vi "SecOverlayParams.vi"(4 "Scan Info":T1, 6 "Time between rf pts\nmicros":dbl, 7 "pixels in y":i16, 9 "c m/s":dbl=1500.0, 10 "Array":i32[](array[numeric]), 11 "pixels in x":i16) -> (0 "scales":cluster{"inc x (mm)":dbl, "inc y (mm)":dbl}, 1 "y scaled":dbl[][](array[numeric]), 2 "x scaled":dbl[][](array[numeric]), 3 "Axis scaling Params":T2 {"Y high" format="%.2f"; "Y low" format="%.2f"; "X left" format="%.2f"; "X right" format="%.2f"})   [LabVIEW 2022 SP3]
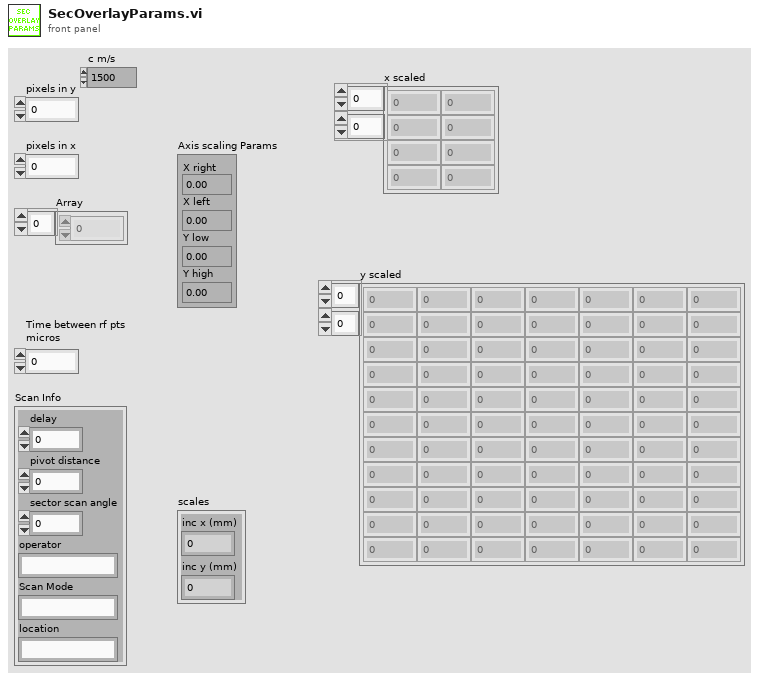
[diagram p1: front panel]
types:
  T1 = cluster{"delay":sgl, "pivot distance":sgl, "sector scan angle":sgl, "operator":string, "Scan Mode":string, "location":string}
  T2 = cluster{"X right":dbl, "X left":dbl, "Y low":dbl, "Y high":dbl}
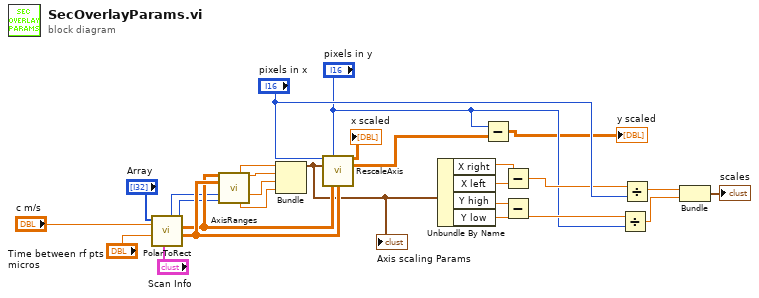
[diagram p0: block diagram]
diagram:
  n1 = call "PolarToRect.vi"("Scan Info"="Scan Info", "Time between pt\nmicros"="Time between rf pts\nmicros", "c m/s"="c m/s", "array dims"="Array") -> ("y"=w9:dbl[][], "x"=w8:dbl[][], "# lines per scan"=w7:u16, "# rf points per line"=w6:u16)  [unwired: 4 out]
  n2 = call "AxisRanges.vi"("x"=w8, "y"=w9, "# rf points per line"=w6, "# lines per scan"=w7) -> ("X right"=w10:dbl, "X left"=w13:dbl, "Y low"=w11:dbl, "Y high"=w12:dbl)  [unwired: 1 in, 7 out]
  n3 = Bundle("X right"=w10, "X left"=w13, "Y low"=w11, "Y high"=w12) -> (w5:T2)  [unwired: 1 out]
  "Axis scaling Params" <- w5
  n4 = call "RescaleAxis.vi"("pixels in x"="pixels in x", "pixels in y"="pixels in y", "Axis scaling Params"=w5, "x"=w8, "y"=w9) -> ("x scaled"=→"x scaled":dbl[][], "y scaled"=w4:dbl[][])  [unwired: 3 in, 6 out]
  n5 = Unbundle By Name(w5) -> ("X right"=w16:dbl, "X left"=w18:dbl, "Y high"=w19:dbl, "Y low"=w17:dbl)
  n6 = Subtract(x="pixels in y", y=w4) -> (x-y=→"y scaled":dbl[][])
  n7 = Subtract(x=w16, y=w18) -> (x-y=w21:dbl)
  n8 = Subtract(x=w19, y=w17) -> (x-y=w20:dbl)
  n9 = Divide(x=w20, y="pixels in y") -> (x/y=w23:dbl)
  n10 = Divide(x=w21, y="pixels in x") -> (x/y=w22:dbl)
  n11 = Bundle(w22, w23) -> (→"scales":cluster{dbl, dbl})  [unwired: 1 in]
